vi "Write Channels_Ref.vi"(8 "error in":errorcluster, 10 "Channels_Ref":refnum<vi>, 11 "Electronic Load in":refnum<class "Electronic Load.lvclass">) -> (0 "error out":errorcluster, 3 "Electronic Load out":refnum<class "Electronic Load.lvclass">)   [LabVIEW 2019, in "Electronic Load.lvlib" / "Electronic Load.lvclass"]
uses:
  Library/Electronic Load.lvclass
  Library/Electronic Load.lvclass/Electronic Load.ctl
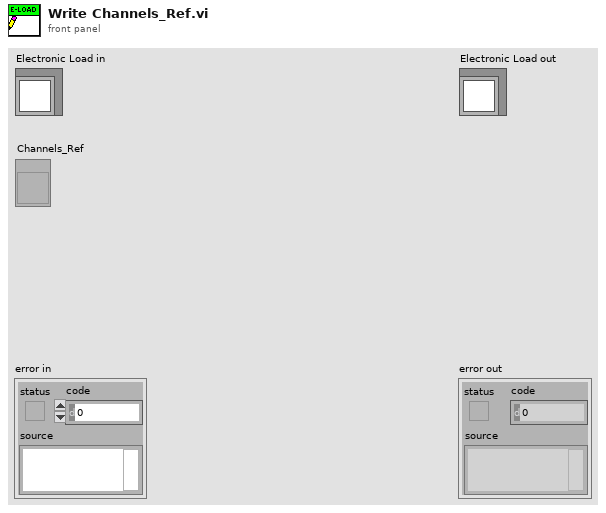
[diagram p1: front panel]
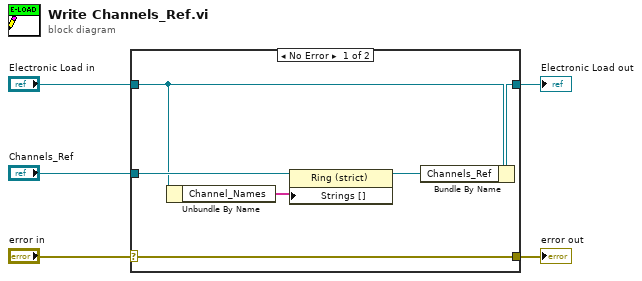
[diagram p0: block diagram]
diagram:
  n1 = case shown="No Error" "error in" {
    selector: "error in" -> [w11 w12]
    tunnel: [w11 w12] -> w4
    tunnel: [w10 w13] -> w2
    tunnel: "Electronic Load in" -> [w7 w13]
    tunnel: "Channels_Ref" -> [w9 _]
    frame No Error {
      n2 = Unbundle By Name(w7) -> ("Channel_Names"=w6:string[])
      n3 = property class="Ring (strict)"(reference=w9, "Strings []"=w6) -> (reference out=w8:refnum<vi>)  [unwired: 1 in, 1 out]
      n4 = Bundle By Name(cluster=w7, "Channels_Ref"=w8) -> (w10:refnum<class "Electronic Load.lvclass">)
    }
    frame Error {
    }
  }
  "error out" <- w4
  "Electronic Load out" <- w2
